vi "MB Modbus Command to Data Unit.vi"(11 "Modbus Command":T1={"Function Code"=1, "Starting Address"=0, "Quantity"=0, "Data"=[], "Discrete"=[]} {"Function Code" items=["Read Coils"=1, "Read Discrete Inputs"=2, "Read Holding Registers"=3, "Read Input Registers"=4, "Write Single Coil"=5, "Write Single Register"=6, "Read Exception Status"=7, "Write Multiple Coils"=15, "Write Multiple Registers"=16]}) -> (3 "Modbus Data Unit":T2={"Function Code"=1, "Data"=[]} {"Function Code" items=["Read Coils"=1, "Read Discrete Inputs"=2, "Read Holding Registers"=3, "Read Input Registers"=4, "Write Single Coil"=5, "Write Single Register"=6, "Read Exception Status"=7, "Write Multiple Coils"=15, "Write Multiple Registers"=16]; "Data" format="%.0x"})   [LabVIEW 2010]
uses:
  MB Modbus Data Unit.ctl
  MB Modbus Command.ctl
panel:
  # "VI Name: MB Command to Data Unit\nPurpose: Creates a Modbus Data Unit based on the user's input."
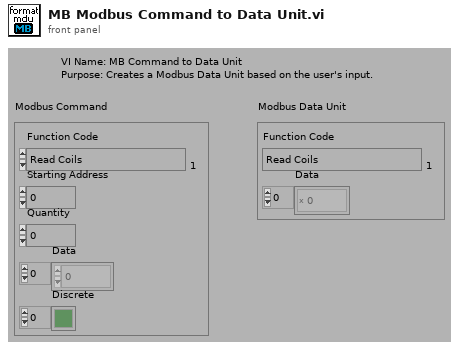
[diagram p1: front panel]
types:
  T1 = typedef "MB Modbus Command.ctl" = cluster{"Function Code":u8, "Starting Address":u16, "Quantity":u16, "Data":u16[], "Discrete":bool[]}
  T2 = typedef "MB Modbus Data Unit.ctl" = cluster{"Function Code":u8, "Data":u8[]}
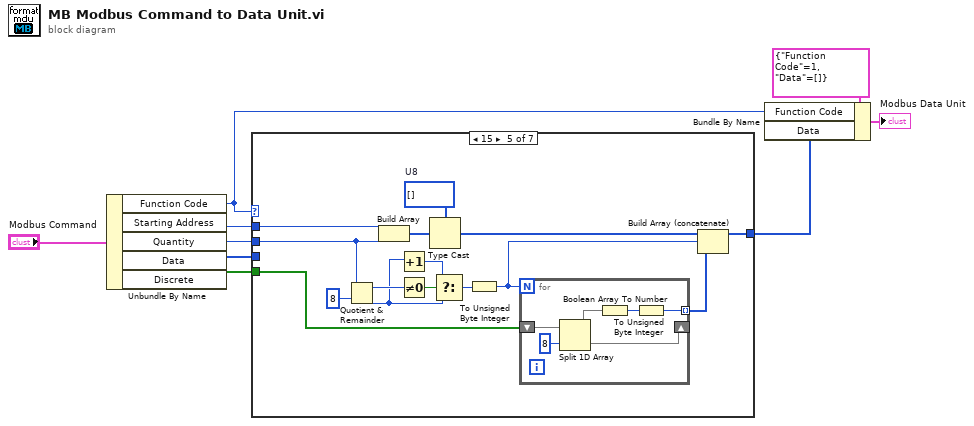
[diagram p0: block diagram]
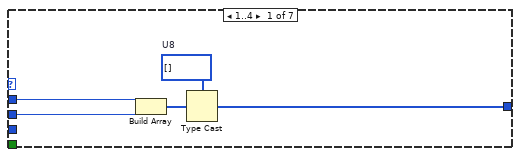
[diagram p2: hidden frame]
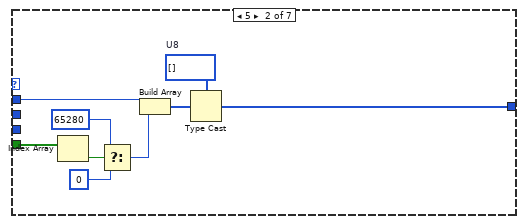
[diagram p3: hidden frame]
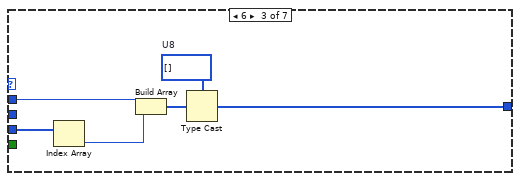
[diagram p4: hidden frame]
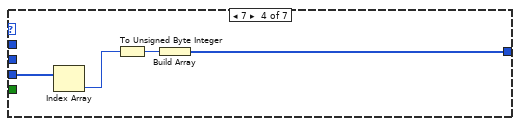
[diagram p5: hidden frame]
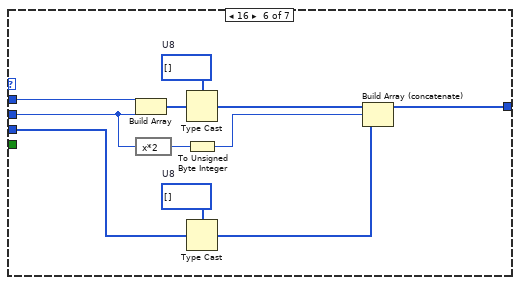
[diagram p6: hidden frame]
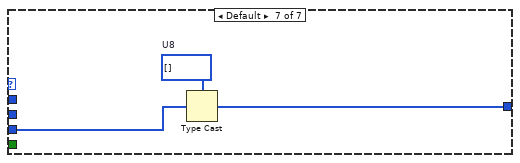
[diagram p7: hidden frame]
diagram:
  n1 = Unbundle By Name("Modbus Command") -> ("Function Code"=w8:u8, "Starting Address"=w7:u16, "Quantity"=w6:u16, "Data"=w5:u16[], "Discrete"=w3:bool[])
  n2 = case shown="15" w8 {
    tunnel: w7 -> [w14 w23 w29 _ w48 w65 _]
    tunnel: w6 -> [w13 _ _ _ w39 w60 _]
    tunnel: w5 -> [_ _ w24 w33 _ w56 w66]
    tunnel: [w10 w20 w26 w30 w38 w61 w67] -> w4
    tunnel: w3 -> [_ w19 _ _ w37 _ _]
    frame 1..4 {
      w11 = u8[] []  # U8
      n3 = Build Array(w14, w13) -> (w12:u16[])
      n4 = Type Cast(type=w11, x=w12) -> (*(type *) &x=w10:u8[])
    }
    frame 5 {
      w21 = u8[] []  # U8
      n5 = Index Array(array=w19) -> (element=w18:bool)  [unwired: 1 in]
      n6 = Select(t=u16 65280, s=w18, f=u16 0) -> (s? t:f=w15:u16)
      n7 = Build Array(w23, w15) -> (w22:u16[])
      n8 = Type Cast(type=w21, x=w22) -> (*(type *) &x=w20:u8[])
    }
    frame 6 {
      w27 = u8[] []  # U8
      n9 = Index Array(array=w24) -> (element=w25:u16)  [unwired: 1 in]
      n10 = Build Array(w29, w25) -> (w28:u16[])
      n11 = Type Cast(type=w27, x=w28) -> (*(type *) &x=w26:u8[])
    }
    frame 7 {
      n12 = Index Array(array=w33) -> (element=w32:u16)  [unwired: 1 in]
      n13 = To Unsigned Byte Integer(number=w32) -> (unsigned 8bit integer=w31:u8)
      n14 = Build Array(w31) -> (w30:u8[])
    }
    frame 15 {
      w46 = u8[] []  # U8
      n15 = Quotient & Remainder(x=w39, y=u16 8) -> (x-y*floor(x/y)=w42:u16, floor(x/y)=w35:u16)
      n16 = Build Array(w48, w39) -> (w47:u16[])
      n17 = Increment(x=w35) -> (x+1=w41:u16)
      n18 = Not Equal To 0?(x=w42) -> (x != 0?=w43:bool)
      n19 = Type Cast(type=w46, x=w47) -> (*(type *) &x=w45:u8[])
      n20 = Select(t=w41, s=w43, f=w35) -> (s? t:f=w40:u16)
      n21 = To Unsigned Byte Integer(number=w40) -> (unsigned 8bit integer=w34:u8)
      n22 = for {
        N: w34 -> [_]
        shift-left: w37 -> [w50]
        shift-right: [w51] -> _
        tunnel: [w53] -> w36 mode=indexing
        n23 = Split 1D Array(array=w50, index=8) -> (first subarray=w52:bool[], second subarray=w51:bool[])
        n24 = Boolean Array To Number(Boolean array=w52) -> (number=w54:u32)
        n25 = To Unsigned Byte Integer(number=w54) -> (unsigned 8bit integer=w53:u8)
      }
      n26 = Build Array (concatenate)(w45, w34, w36) -> (w38:u8[])
    }
    frame 16 {
      w57 = u8[] []  # U8
      w63 = u8[] []  # U8
      n27 = Build Array(w65, w60) -> (w64:u16[])
      n28 = expression code="x*2"(w60) -> (w59:u16)
      n29 = Type Cast(type=w63, x=w64) -> (*(type *) &x=w62:u8[])
      n30 = To Unsigned Byte Integer(number=w59) -> (unsigned 8bit integer=w58:u8)
      n31 = Type Cast(type=w57, x=w56) -> (*(type *) &x=w55:u8[])
      n32 = Build Array (concatenate)(w62, w58, w55) -> (w61:u8[])
    }
    frame Default {
      w68 = u8[] []  # U8
      n33 = Type Cast(type=w68, x=w66) -> (*(type *) &x=w67:u8[])
    }
  }
  n34 = Bundle By Name(cluster=T2 {"Function Code"=1, "Data"=[]} ("MODBUS Data Unit"), "Function Code"=w8, "Data"=w4) -> (→"Modbus Data Unit":T2)
